vi "PicoScope4000aGetTimebase2.vi"(4 "Number of Samples":u32, 6 "Memory Segment":u32, 7 "Acquisition Settings":T1={"preTriggerSamples"=0, "postTriggerSamples"=5000000, "timebase"=5} {"postTriggerSamples" format="%_6p"; "preTriggerSamples" format="%_6p"}, 8 "error in (no error)":errorcluster, 11 "handle in":i16) -> (0 "error out":errorcluster, 3 "handle out":i16, 5 "Properties Panel":T2={"Sample Frequency"=41666668.0, "Sample Rate"=2.4000000209412065e-08, "Max Samples Available"=26843008, "Number of Samples"=0, "Total Capture Time (sec) "=0.0, "Max Total Capture Time Available (sec)"=0.6442322134971619} {"Max Total Capture Time Available (sec)" format="%.3p"; "Sample Frequency" format="%.6p"; "Sample Rate" format="%.3p"; "Max Samples Available" format="%_6p"; "Total Capture Time (sec)" format="%.3p"})   [LabVIEW 2010]
doc: "Calls Gettimebase function"
uses:
  Program Files/Pico Technology/SDK/lib/ps4000a.dll
  shared/Acquisition Settings.ctl
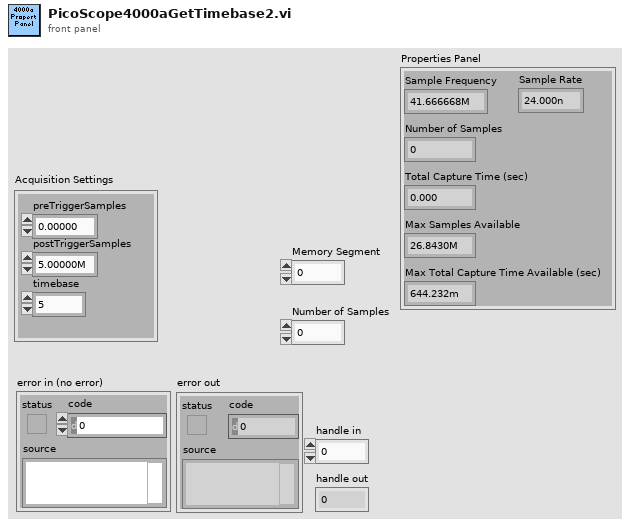
[diagram p1: front panel]
types:
  T1 = typedef "Acquisition Settings.ctl" = cluster{"preTriggerSamples":u64, "postTriggerSamples":u64, "timebase":u32}
  T2 = cluster{"Sample Frequency":dbl, "Sample Rate":dbl, "Max Samples Available":u64, "Number of Samples":u64, "Total Capture Time (sec) ":dbl, "Max Total Capture Time Available (sec)":dbl}
  T3 = cluster{sgl, sgl, "maxSamples":i32, "Number of Samples":u32, sgl, sgl}
  T4 = cluster{dbl, dbl, "maxSamples":i32, "Number of Samples":u32, dbl, dbl}
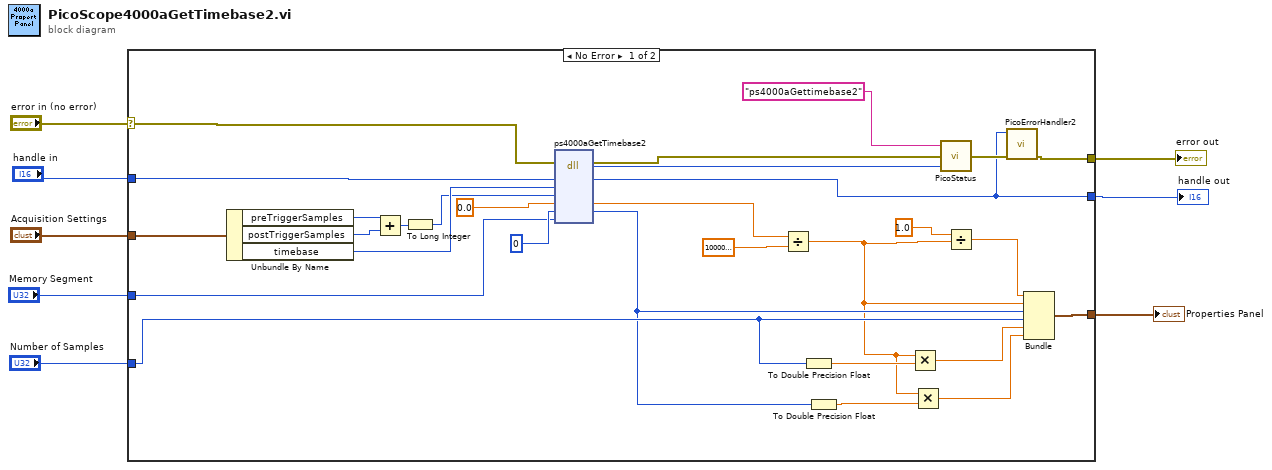
[diagram p0: block diagram]
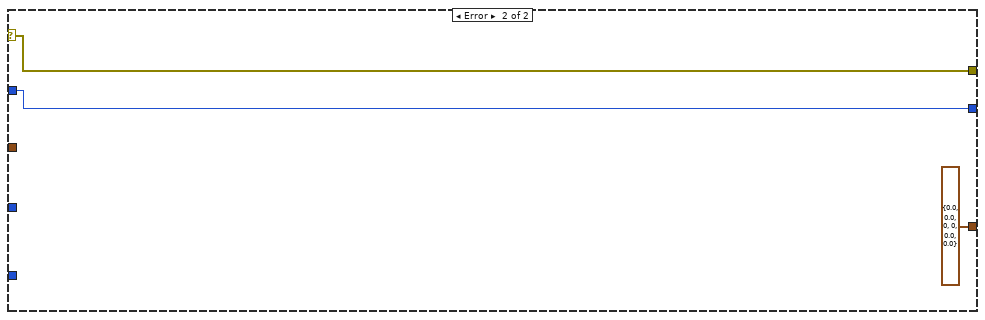
[diagram p2: hidden frame]
diagram:
  n1 = case shown="No Error" "error in (no error)" {
    selector: "error in (no error)" -> [w15 w40]
    tunnel: [w13 w40] -> w8
    tunnel: [w12 w39] -> w7
    tunnel: "Memory Segment" -> [w27 _]
    tunnel: "Number of Samples" -> [w23 _]
    tunnel: "handle in" -> [w26 w39]
    tunnel: [w19 T3 {0.0, 0.0, "maxSamples"=0, "Number of Samples"=0, 0.0, 0.0}] -> w2
    tunnel: "Acquisition Settings" -> [w9 _]
    frame No Error {
      n2 = Unbundle By Name(w9) -> ("preTriggerSamples"=w32:u64, "postTriggerSamples"=w33:u64, "timebase"=w34:u32)
      n3 = Add(x=w32, y=w33) -> (x+y=w11:u64)
      n4 = To Long Integer(number=w11) -> (32bit integer=w10:i32)
      n5 = dll-call lib="/Program Files/Pico Technology/SDK/lib/ps4000a.dll" fn="ps4000aGetTimebase2"(error in=w15, "handle"=w26, "timebase"=w34, "noSamples"=w10, "timeIntervalNanoseconds"=sgl 0.0, "maxSamples"=0, "segmentIndex"=w27) -> (error out=w35:errorcluster, "PICO_STATUS"=w28:u32, "handle"=w12:i16, "timeIntervalNanoseconds"=w36:sgl, "maxSamples"=w21:i32)  [unwired: 5 in, 1 out]
      n6 = Divide(x=w36, y=1000000000.0) -> (x/y=w18:dbl)
      n7 = To Double Precision Float(number=w23) -> (double precision float=w25:dbl)
      n8 = To Double Precision Float(number=w21) -> (double precision float=w22:dbl)
      n9 = Multiply(x=w18, y=w25) -> (x*y=w24:dbl)
      n10 = Multiply(x=w18, y=w22) -> (x*y=w20:dbl)
      n11 = call "PicoStatus.vi"("PICO STATUS"=w28, "error in"=w35, "source"="ps4000aGettimebase2") -> ("error out"=w14:errorcluster)
      n12 = Divide(x=1.0, y=w18) -> (x/y=w16:dbl)
      n13 = call "PicoErrorHandler2.vi"("error in (no error)"=w14, "handle In"=w12) -> ("error out"=w13:errorcluster)  [unwired: 9 in]
      n14 = Bundle(w16, w18, "maxSamples"=w21, "Number of Samples"=w23, w24, w20) -> (w19:T4)  [unwired: 1 in]
    }
    frame Error {
    }
  }
  "error out" <- w8
  "handle out" <- w7
  "Properties Panel" <- w2
